vi "testItemInfoGet.vi"(8 "error in (no error)":errorcluster caption="error in", 11 "basePath":path) -> (0 "error out":errorcluster, 1 "TDD":T1, 2 "xml_detail":T2, 3 "singleItemInfo":T3[](array[typedef]))   [LabVIEW 2011]
uses:
  dataType/sSpec.ctl
  dataType/xml_detail.ctl
  dataType/TDD.ctl
  32port/subvi/dataType/HW_xml.ctl
  32port/subvi/dataType/singleTestParameter.ctl
  32port/subvi/dataType/cluResult.ctl
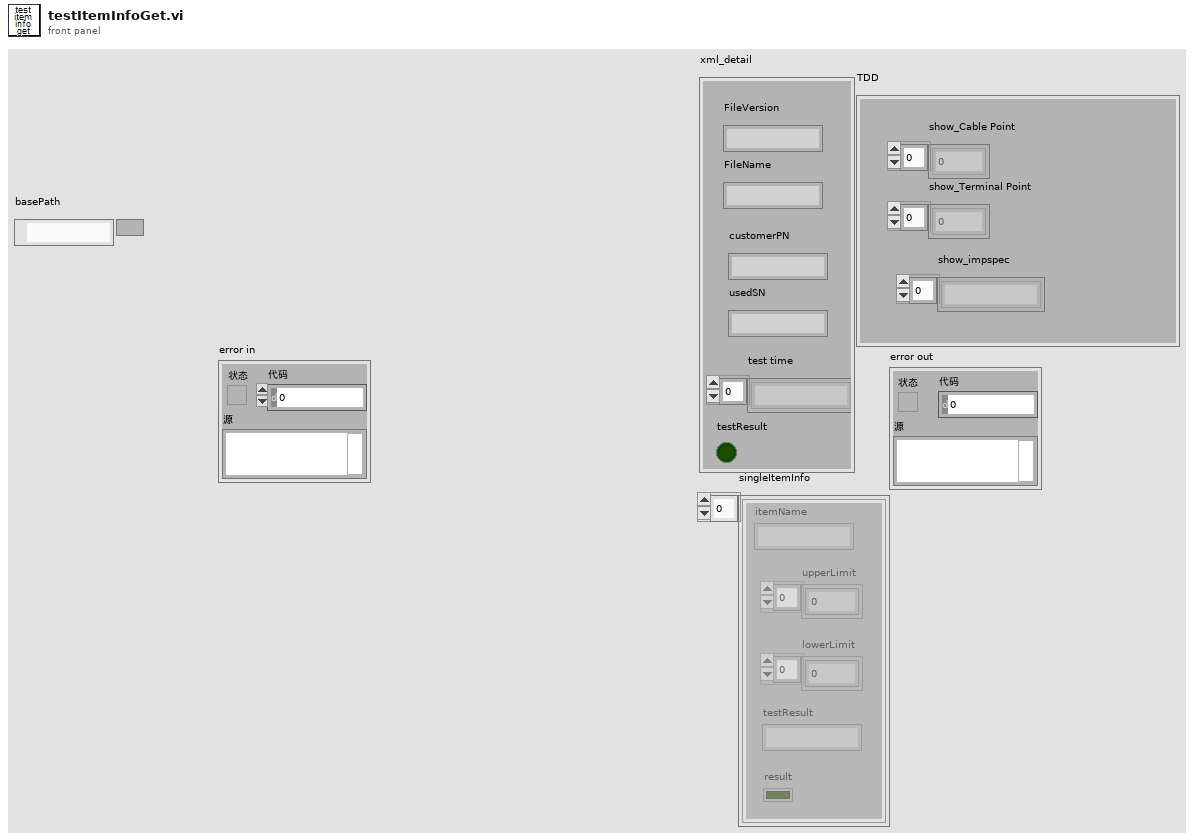
[diagram p1: front panel]
types:
  T1 = typedef "TDD.ctl" = cluster{"show_Cable Point":dbl[], "show_Terminal Point":dbl[], "show_impspec":string[]}
  T2 = typedef "xml_detail.ctl" = cluster{"FileVersion":string, "FileName":string, "customerPN":string, "usedSN":string, "test time":string[], "testResult":bool}
  T3 = typedef "sSpec.ctl" = cluster{"itemName":string, "upperLimit":dbl[], "lowerLimit":dbl[], "testResult":string, "result":bool}
  T4 = cluster{"FileVersion":string, "FileName":string, "test time":string[], "original Path":path, "show_TDD11":string[], "show_TDD22":string[], "show_impspec":string[], "usedSN":string, "diffspec":cluster{"limit Spec":dbl[][], "Diff Test Item Name":string[], "Spec _Col":i32[]}, "secondresult":bool[], "show_Terminal Point":dbl[], "show_Cable Point":dbl[], "customerPN":string, "auto get refer point":bool, "width1":i32, "width2":i32}
  T5 = cluster{"limit Spec":dbl[][], "Diff Test Item Name":string[], "Spec _Col":i32[]}
  T6 = cluster{"swapped test item name":string[], "secondresult":bool[]}
  T7 = typedef "HW_xml.ctl" = cluster{"FileVersion":string, "FileName":string, "test time":string[], "original Path":path, "show_impspec":string[], "usedSN":string, "show_Terminal Point":dbl[], "show_Cable Point":dbl[], "sSpec":T8[], "resultCluster":T9, "customerPN":string}
  T8 = typedef "singleTestParameter.ctl" = cluster{"itemName":string, "testPair":dbl, "chartDisplay?":bool, "spec":cluster{"upper limit":cluster{"dx":dbl[], "dy":dbl[]}, "lowwer limit":cluster{"dx":dbl[], "dy":dbl[]}}, "smooth":cluster{"smooth?":bool, "smoothPoints":dbl}, "Compensation(ohm)":dbl, "Filter Risetime(ps)":dbl, "singlePoint":string[], "offset":dbl[], "Skew max(ps)":dbl}
  T9 = typedef "cluResult.ctl" = cluster{"itemResult":string[], "itemName":string[]}
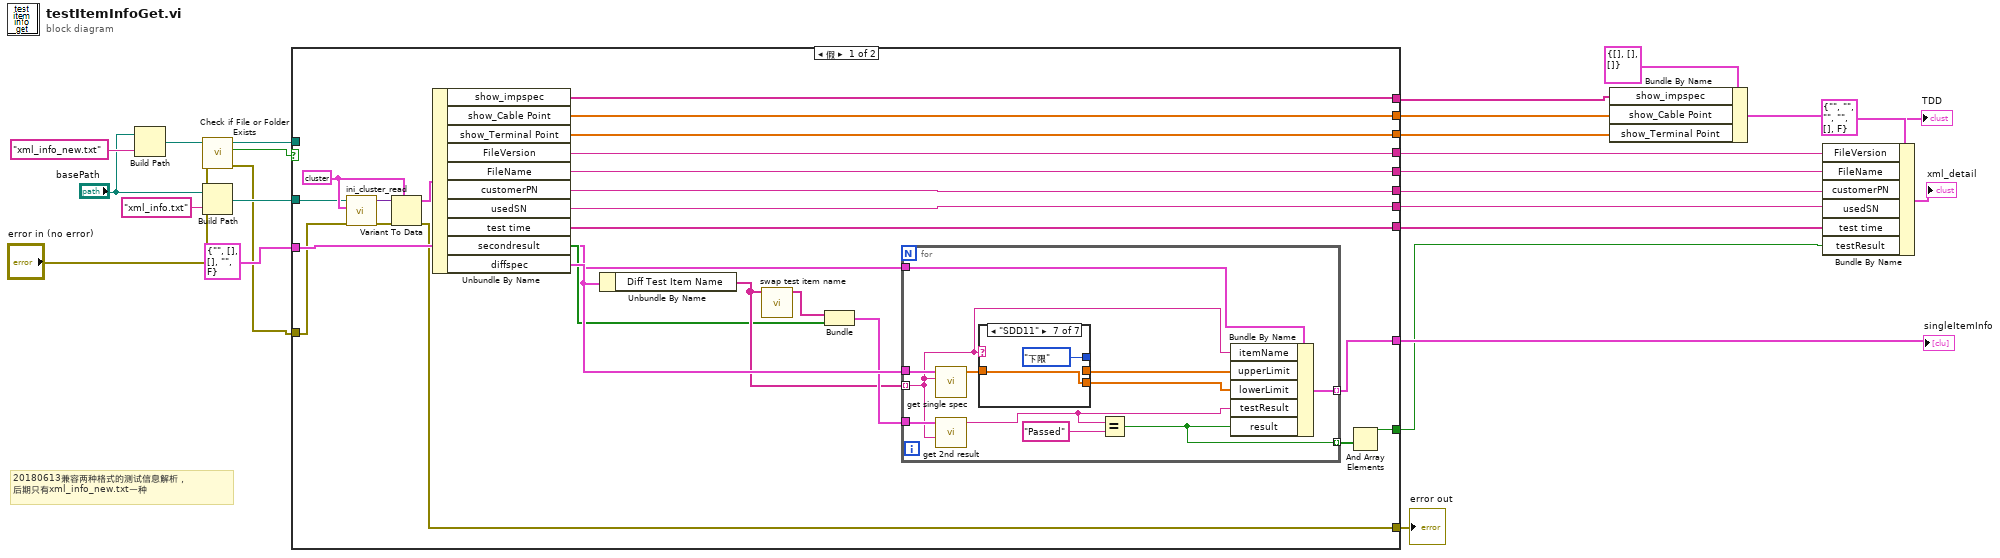
[diagram p0: block diagram]
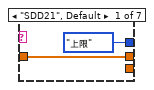
[diagram p2: hidden frame]
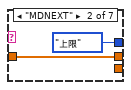
[diagram p3: hidden frame]
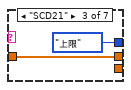
[diagram p4: hidden frame]
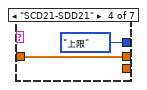
[diagram p5: hidden frame]
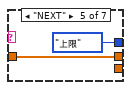
[diagram p6: hidden frame]
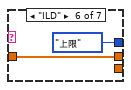
[diagram p7: hidden frame]
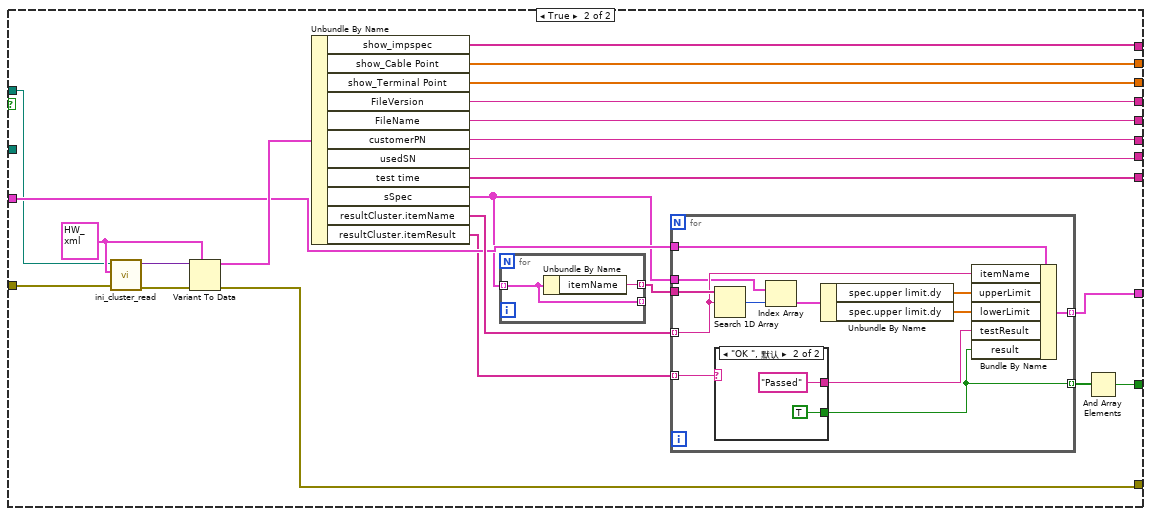
[diagram p8: hidden frame]
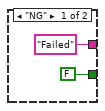
[diagram p9: hidden frame]
diagram:
  # "20180613兼容两种格式的测试信息解析，\n后期只有xml_info_new.txt一种"
  n1 = Build Path(base path="basePath", name or relative path="xml_info_new.txt" ("名称或相对路径")) -> (appended path=w21:path)
  n2 = call <vilib>:"Check if File or Folder Exists.vi"("error in (no error)"="error in (no error)", "path"=w21) -> ("error out"=w2:errorcluster, "file or folder exists?"=w19:bool, "dup path"=w20:path)  [unwired: 7 in]
  n3 = Build Path(base path="basePath", name or relative path="xml_info.txt" ("名称或相对路径")) -> (appended path=w18:path)
  n4 = case shown="假" w19 {
    tunnel: T3 {"itemName"="", "upperLimit"=[], "lowerLimit"=[], "testResult"="", "result"=FALSE} ("sSpec") -> [w41 w93]
    tunnel: w20 -> [_ w89]
    tunnel: [w39 w88] -> w17
    tunnel: w18 -> [w40 _]
    tunnel: [w38 w87] -> w7
    tunnel: [w37 w86] -> w6
    tunnel: [w36 w85] -> w16
    tunnel: [w35 w84] -> w15
    tunnel: [w31 w80] -> w11
    tunnel: [w34 w83] -> w14
    tunnel: [w33 w82] -> w13
    tunnel: [w32 w81] -> w8
    tunnel: [w30 w78] -> w4
    tunnel: w2 -> [w28 w77]
    tunnel: [w26 w75] -> w1
    frame False {
      w43 = T4 {"FileVersion"="DevelopmentSystem", "FileName"="DevelopmentSystem", "test time"=["2016/11/14 11:59:03"], "original Path"=path "D:/高频房软件/2. HPTS_VNA_Rev2.7.1.3-1107最新源码/Demo_data", "show_TDD11"=[], "show_TDD22"=[], "show_impspec"=[], "usedSN"="", "diffspec"={"limit Spec"=[], "Diff Test Item Name"=[], "Spec _Col"=[]}, "secondresult"=[], "show_Terminal Point"=[], "show_Cable Point"=[], "customerPN"="", "auto get refer point"=FALSE, "width1"=0, "width2"=0} ("xml_info")
      n5 = call "ini_cluster_read.vi"("error in (no error)"=w28, "INI Fomatted Cluster Type"=w43, "configuration file path"=w40) -> ("error out"=w27:errorcluster, "ini cluster out"=w42:variant)  [unwired: 7 in]
      n6 = Variant To Data(error in=w27, type=w43, Variant=w42) -> (data=w44:T4, error out=w26:errorcluster)
      n7 = Unbundle By Name(w44) -> ("show_impspec"=w32:string[], "show_Cable Point"=w38:dbl[], "show_Terminal Point"=w37:dbl[], "FileVersion"=w36:string, "FileName"=w35:string, "customerPN"=w34:string, "usedSN"=w33:string, "test time"=w31:string[], "secondresult"=w46:bool[], "diffspec"=w49:T5)
      n8 = Unbundle By Name(w49) -> ("Diff Test Item Name"=w47:string[])
      n9 = call "swap test item name.vi"("Diff Test Item Name"=w47) -> ("swapped test item name"=w45:string[])  [unwired: 10 in]
      n10 = Bundle("swapped test item name"=w45, "secondresult"=w46) -> (w48:T6)  [unwired: 1 in]
      n11 = for {
        tunnel: w47 -> [w57] mode=indexing
        tunnel: w41 -> [w60]
        tunnel: w48 -> [w59]
        tunnel: w49 -> [w58]
        tunnel: [w53] -> w39 mode=indexing
        tunnel: [w50] -> w29 mode=indexing
        n12 = call "get single spec.vi"("single item name"=w57, "single spec"=w58) -> ("single spec"=w56:dbl[])  [unwired: 9 in]
        n13 = call "get 2nd result.vi"("test item"=w57, "itemClusters"=w59) -> ("result string"=w52:string)  [unwired: 9 in]
        n14 = case shown="\"SDD11\"" w57 {
          tunnel: [enum16{"上限", "下限"}."上限" ("limit type") enum16{"上限", "下限"}."上限" ("limit type") enum16{"上限", "下限"}."上限" ("limit type") enum16{"上限", "下限"}."上限" ("limit type") enum16{"上限", "下限"}."上限" ("limit type") enum16{"上限", "下限"}."上限" ("limit type") enum16{"上限", "下限"}."下限" ("limit type")] -> _
          tunnel: w56 -> [w61 w63 w65 w67 w69 w71 w73]
          tunnel: [w61 w63 w65 w67 w69 w71 _] -> w55
          tunnel: [_ _ _ _ _ _ w73] -> w54
          frame "SDD21", Default {
          }
          frame "MDNEXT" {
          }
          frame "SCD21" {
          }
          frame "SCD21-SDD21" {
          }
          frame "NEXT" {
          }
          frame "ILD" {
          }
          frame "SDD11" {
          }
        }
        n15 = Equal?(x=w52, y="Passed") -> (x = y?=w50:bool)
        n16 = Bundle By Name(cluster=w60, "itemName"=w57, "upperLimit"=w55, "lowerLimit"=w54, "testResult"=w52, "result"=w50) -> (w53:T3)
      }
      n17 = And Array Elements(Boolean array=w29) -> (logical AND=w30:bool)
    }
    frame True {
      w96 = T7 {"FileVersion"="DevelopmentSystem", "FileName"="DevelopmentSystem", "test time"=["2016/11/14 11:59:03"], "original Path"=path "D:/高频房软件/2. HPTS_VNA_Rev2.7.1.3-1107最新源码/Demo_data", "show_impspec"=[], "usedSN"="", "show_Terminal Point"=[], "show_Cable Point"=[], "sSpec"=[], "resultCluster"={"itemResult"=[], "itemName"=[]}, "customerPN"=""} ("xml_info")
      n18 = call "ini_cluster_read.vi"("error in (no error)"=w77, "INI Fomatted Cluster Type"=w96, "configuration file path"=w89) -> ("error out"=w76:errorcluster, "ini cluster out"=w97:variant)  [unwired: 7 in]
      n19 = Variant To Data(error in=w76, type=w96, Variant=w97) -> (data=w95:T7, error out=w75:errorcluster)
      n20 = Unbundle By Name(w95) -> ("show_impspec"=w81:string[], "show_Cable Point"=w87:dbl[], "show_Terminal Point"=w86:dbl[], "FileVersion"=w85:string, "FileName"=w84:string, "customerPN"=w83:string, "usedSN"=w82:string, "test time"=w80:string[], "sSpec"=w90:T8[], "resultCluster.itemName"=w94:string[], "resultCluster.itemResult"=w92:string[])
      n21 = for {
        tunnel: [w99] -> _ mode=indexing
        tunnel: w90 -> [w99] mode=indexing
        tunnel: [w98] -> w91 mode=indexing
        n22 = Unbundle By Name(w99) -> ("itemName"=w98:string)
      }
      n23 = for {
        tunnel: w94 -> [w109] mode=indexing
        tunnel: w93 -> [w111]
        tunnel: w92 -> [w102] mode=indexing
        tunnel: w91 -> [w110]
        tunnel: w90 -> [w108]
        tunnel: [w103] -> w88 mode=indexing
        tunnel: [w100] -> w79 mode=indexing
        n24 = Search 1D Array(1D array=w110, element=w109) -> (index of element=w107:i32)  [unwired: 1 in]
        n25 = case shown="\"OK \", 默认" w102 {
          tunnel: ["Failed" "Passed"] -> w101
          tunnel: [FALSE TRUE] -> w100
          frame "NG" {
          }
          frame "OK ", Default {
          }
        }
        n26 = Index Array(array=w108, index=w107) -> (element=w106:T8)
        n27 = Unbundle By Name(w106) -> ("spec.upper limit.dy"=w105:dbl[], "spec.upper limit.dy"=w104:dbl[])
        n28 = Bundle By Name(cluster=w111, "itemName"=w109, "upperLimit"=w105, "lowerLimit"=w104, "testResult"=w101, "result"=w100) -> (w103:T3)
      }
      n29 = And Array Elements(Boolean array=w79) -> (logical AND=w78:bool)
    }
  }
  "singleItemInfo" <- w17
  "error out" <- w1
  n30 = Bundle By Name(cluster=T1 {"show_Cable Point"=[], "show_Terminal Point"=[], "show_impspec"=[]} ("簇"), "show_impspec"=w8, "show_Cable Point"=w7, "show_Terminal Point"=w6) -> (→"TDD":T1)
  n31 = Bundle By Name(cluster=T2 {"FileVersion"="", "FileName"="", "customerPN"="", "usedSN"="", "test time"=[], "testResult"=FALSE} ("xml_detail"), "FileVersion"=w16, "FileName"=w15, "customerPN"=w14, "usedSN"=w13, "test time"=w11, "testResult"=w4) -> (→"xml_detail":T2)
